vi "Zero Crossing Detector.vi"(8 "Direction":enum16{"Rising", "Falling"}(ring)=enum."Falling", 9 "offset":u64, 10 "Y":dbl[](array[numeric])) -> (3 "X":i32)   [LabVIEW 2017]
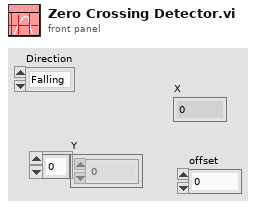
[diagram p1: front panel]
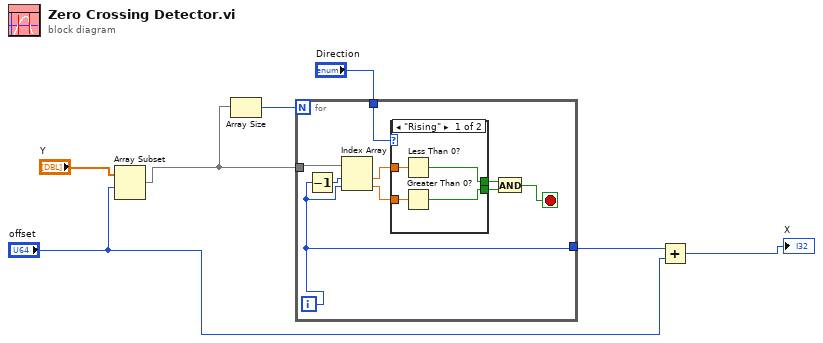
[diagram p0: block diagram]
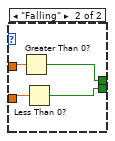
[diagram p2: hidden frame]
diagram:
  n1 = Array Subset(array="Y", index="offset") -> (w4:dbl[])  [unwired: 1 in]
  n2 = Array Size(array=w4) -> (size(s)=w7:i32)
  n3 = for {
    N: w7 -> [_]
    tunnel: w4 -> [w16]
    tunnel: [w14] -> w3
    tunnel: "Direction" -> [w8]
    i -> [w14]
    stop <- w11 stop-if-true
    n4 = Decrement(x=w14) -> (x-1=w15:i32)
    n5 = Index Array(array=w16, index #1=w15, index #2=w14) -> (element #1=w13:dbl, element #2=w12:dbl)
    n6 = case shown="\"Rising\"" w8 {
      tunnel: w13 -> [w20 w24]
      tunnel: w12 -> [w19 w22]
      tunnel: [w18 w23] -> w10
      tunnel: [w17 w21] -> w9
      frame "Rising" {
        n7 = Less Than 0?(x=w20) -> (x < 0?=w18:bool)
        n8 = Greater Than 0?(x=w19) -> (x > 0?=w17:bool)
      }
      frame "Falling" {
        n9 = Greater Than 0?(x=w24) -> (x > 0?=w23:bool)
        n10 = Less Than 0?(x=w22) -> (x < 0?=w21:bool)
      }
    }
    n11 = And(x=w10, y=w9) -> (x .and. y?=w11:bool)
  }
  n12 = Add(x=w3, y="offset") -> (x+y=→"X":u64)
